vi "Unbunde bundle interface clusters for PI Terminal.vi"(0 "System No.":i32=1 min=1 max=4 step=1, 3 "Interface configuration":T9(array[cluster])=[{"RS232 portnumber"=0, "Timeout"=1000, "RS232 baud rate"=57600, "Interface"=0, "GPIB Bus"=0, "GPIB address"=4, "GPIB mode"=0}] {"Interface" items=["RS232", "GPIB", "DLL", "TCP-IP", "USB", "Analog"]; "RS232 portnumber" items=["COM1", "COM2", "COM3", "COM4", "COM5", "COM6", "COM7", "COM8", "COM9", "COM10", "COM11", "COM12", "COM13", "COM14", "COM15", "COM16", "COM17", "COM18", "COM19", "COM20", "COM21", "COM22", "COM23", "COM24", "COM25", "COM26", "COM27", "COM28", "COM29", "COM30"]}, 6 "DLL Interface\nconfiguration":T7(array[cluster])=[{"DLL for Device"=0, "DLL interface"=2, "Parameter"="1"}] {"DLL for Device" items=["C-843", "C-844", "E-710", "C-843.PM", "C-865", "E-761", "Mercury", "E-755", "E-753", "C-866", "E-712", "E-725", "E-861", "C-867", "E-517", "E-816", "E-709", "PI_GCS2_DLL", "HydraPollux"]; "DLL interface" items=["RS232", "GPIB", "Board", "TCP-IP", "USB", "RS232_DC", "USB_DC", "TCPIP_DC"]}, 7 "TCP/IP Configuration":T4(array[cluster])=[{"Host address/name"="localhost", "Port"=3000, "Board"=0}, {"Host address/name"="localhost", "Port"=3000, "Board"=0}, {"Host address/name"="localhost", "Port"=3000, "Board"=0}, {"Host address/name"="localhost", "Port"=3000, "Board"=0}], 9 "Flow control":T5(array[cluster])=[{"input XON/XOFF"=FALSE, "input HW Handshake"=FALSE, "input alt HW HShk"=FALSE, "output XON/XOFF"=FALSE, "output HW Handshake"=FALSE, "output alt HW HShk"=FALSE, "XOFF byte "=19, "XON byte"=17, "parity error byte"=0}, {"input XON/XOFF"=FALSE, "input HW Handshake"=FALSE, "input alt HW HShk"=FALSE, "output XON/XOFF"=FALSE, "output HW Handshake"=FALSE, "output alt HW HShk"=FALSE, "XOFF byte "=19, "XON byte"=17, "parity error byte"=0}, {"input XON/XOFF"=FALSE, "input HW Handshake"=FALSE, "input alt HW HShk"=FALSE, "output XON/XOFF"=FALSE, "output HW Handshake"=FALSE, "output alt HW HShk"=FALSE, "XOFF byte "=19, "XON byte"=17, "parity error byte"=0}, {"input XON/XOFF"=FALSE, "input HW Handshake"=FALSE, "input alt HW HShk"=FALSE, "output XON/XOFF"=FALSE, "output HW Handshake"=FALSE, "output alt HW HShk"=FALSE, "XOFF byte "=19, "XON byte"=17, "parity error byte"=0}] {"parity error byte" format="%.0x"; "XON byte" format="%.0x"; "XOFF byte" format="%.0x"}, 10 "Termination character":T3[](array[typedef])=[enum."LF", enum."LF", enum."LF", enum."LF"]) -> (12 "Term.char":T3, 13 "TCP/IP Config. System":T2={"Host address/name"="localhost", "Port"=3000, "Board"=0, "Timeout"=5000}, 14 "Interface":T8 items=["RS232", "GPIB", "DLL", "TCP-IP", "USB", "Analog"], 15 "RS232 configuration system":T11 {"Handshake" items=["None", "HW", "XON/XOFF"]; "Portnumber" items=["COM 1", "COM 2", "COM 3", "COM 4", "COM 5", "COM 6", "COM 7", "COM 8", "COM 9", "COM 10", "COM 11", "COM 12", "COM 13", "COM 14", "COM 15", "COM 16", "COM 17", "COM 18", "COM 19", "COM 20", "COM 21", "COM 22", "COM 23", "COM 24", "COM 25", "COM 26", "COM 27", "COM28", "COM 29", "COM 30"]}, 16 "GPIB configuration system":T10, 17 "DLL for Device":T1 items=["C-843", "C-844", "E-710", "C-843.PM", "C-865", "E-761", "Mercury", "E-755", "E-753", "C-866", "E-712", "E-725", "E-861", "C-867", "E-517", "E-816", "E-709", "PI_GCS2_DLL", "HydraPollux"], 18 "DLL interface":T6 items=["RS232", "GPIB", "Board", "TCP-IP", "USB", "RS232_DC", "USB_DC", "TCPIP_DC"])   [LabVIEW 2020]
doc: "This VI is a sub-VI for PI Terminal.vi. It unbundles Interface configuration and DLL Interface configuration and returns the cluster contents in a different composition which is used by PI Terminal.vi."
uses:
  Available DLL interfaces.ctl
  Available interfaces.ctl
  Available DLLs.ctl
  Termination character.ctl
panel:
  # "This vi is a sub-vi for\" PI Terminal.vi\". It unbundles \"Interface configuration\" and \"DLL Interface configuration\" and returns the cluster contents in different composition which is used by \"PI Terminal.vi\" ."
  # "Output:"
  # "TCP/IP:"
  # "DLL:"
  # "General:"
  # "RS232:"
  # "GPIB:"
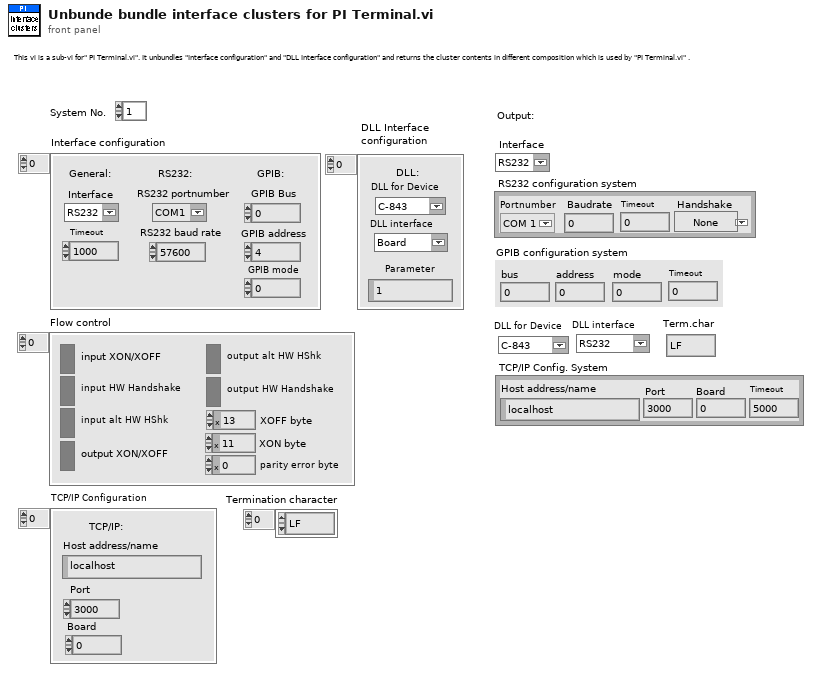
[diagram p1: front panel]
types:
  T1 = typedef "Available DLLs.ctl" = u16
  T2 = cluster{"Host address/name":string, "Port":i32, "Board":i32, "Timeout":i32}
  T3 = typedef "Termination character.ctl" = enum16{"LF", "CR", "LFCR", "CRLF"}
  T4 = cluster{"Host address/name":string, "Port":i32, "Board":i32}[]
  T5 = cluster{"input XON/XOFF":bool, "input HW Handshake":bool, "input alt HW HShk":bool, "output XON/XOFF":bool, "output HW Handshake":bool, "output alt HW HShk":bool, "XOFF byte ":u8, "XON byte":u8, "parity error byte":u16}[]
  T6 = typedef "Available DLL interfaces.ctl" = u16
  T7 = cluster{"DLL for Device":T1, "DLL interface":T6, "Parameter":string}[]
  T8 = typedef "Available interfaces.ctl" = u16
  T9 = cluster{"RS232 portnumber":u16, "Timeout":i32, "RS232 baud rate":u32, "Interface":T8, "GPIB Bus":i16, "GPIB address":i16, "GPIB mode":i16}[]
  T10 = cluster{"bus":i16, "address":i16, "mode":i16, "Timeout":i32}
  T11 = cluster{"Portnumber":u32, "Timeout":i32, "Baudrate":u32, "Handshake":u16}
  T12 = cluster{"Host address/name":string, "Port":i32, "Board":i32}
  T13 = cluster{"input XON/XOFF":bool, "input HW Handshake":bool, "input alt HW HShk":bool, "output XON/XOFF":bool, "output HW Handshake":bool, "output alt HW HShk":bool, "XOFF byte ":u8, "XON byte":u8, "parity error byte":u16}
  T14 = cluster{"RS232 portnumber":u16, "Timeout":i32, "RS232 baud rate":u32, "Interface":T8, "GPIB Bus":i16, "GPIB address":i16, "GPIB mode":i16}
  T15 = cluster{"DLL for Device":T1, "DLL interface":T6, "Parameter":string}
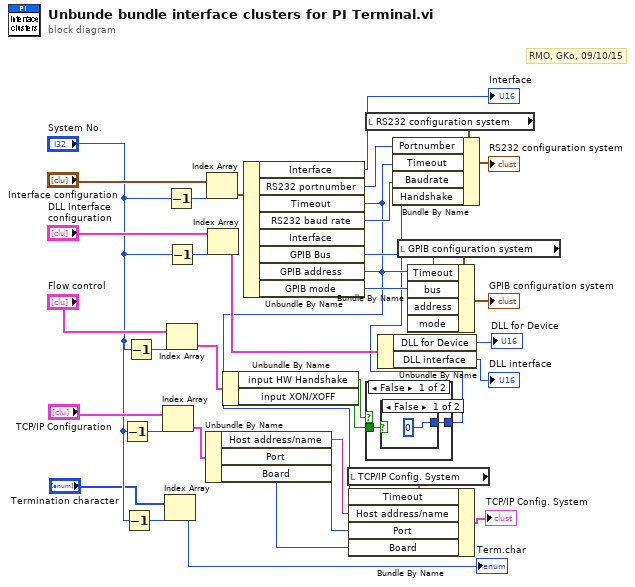
[diagram p0: block diagram]
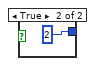
[diagram p2: hidden frame]
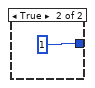
[diagram p3: hidden frame]
diagram:
  # "RMO, GKo, 09/10/15"
  n1 = Decrement(x="System No.") -> (x-1=w14:i32)
  n2 = Decrement(x="System No.") -> (x-1=w12:i32)
  n3 = Decrement(x="System No.") -> (x-1=w19:i32)
  n4 = Index Array(array="TCP/IP Configuration", index=w14) -> (element=w8:T12)
  n5 = Index Array(array="Termination character", index=w12) -> (element=→"Term.char":T3)
  n6 = Decrement(x="System No.") -> (x-1=w35:i32)
  n7 = Decrement(x="System No.") -> (x-1=w36:i32)
  n8 = Index Array(array="Flow control", index=w19) -> (element=w18:T13)
  n9 = Unbundle By Name(w8) -> ("Host address/name"=w5:string, "Port"=w4:i32, "Board"=w3:i32)
  n10 = Index Array(array="Interface configuration", index=w35) -> (element=w29:T14)
  n11 = Index Array(array="DLL Interface\nconfiguration", index=w36) -> (element=w37:T15)
  n12 = Unbundle By Name(w18) -> ("input HW Handshake"=w17:bool, "input XON/XOFF"=w16:bool)
  n13 = Unbundle By Name(w29) -> ("Interface"=→"Interface":T8, "RS232 portnumber"=w30:u16, "Timeout"=w6:i32, "RS232 baud rate"=w31:u32, "GPIB Bus"=w32:i16, "GPIB address"=w33:i16, "GPIB mode"=w34:i16)  [unwired: 1 out]
  n14 = local read "TCP/IP Config. System"() -> (w7:T2)
  n15 = Bundle By Name(cluster=w7, "Timeout"=w6, "Host address/name"=w5, "Port"=w4, "Board"=w3) -> (→"TCP/IP Config. System":T2)
  n16 = local read "RS232 configuration system"() -> (w28:T11)
  n17 = case shown="False" w17 {
    tunnel: w16 -> [w39 _]
    tunnel: [w38 1] -> w15
    frame False {
      n18 = case shown="False" w39 {
        tunnel: [0 2] -> w38
        frame False {
        }
        frame True {
        }
      }
    }
    frame True {
    }
  }
  n19 = Unbundle By Name(w37) -> ("DLL for Device"=→"DLL for Device":T1, "DLL interface"=→"DLL interface":T6)
  n20 = Bundle By Name(cluster=w28, "Portnumber"=w30, "Timeout"=w6, "Baudrate"=w31, "Handshake"=w15) -> (→"RS232 configuration system":T11)
  n21 = local read "GPIB configuration system"() -> (w26:T10)
  n22 = Bundle By Name(cluster=w26, "Timeout"=w6, "bus"=w32, "address"=w33, "mode"=w34) -> (→"GPIB configuration system":T10)
